vi "Get comma separated item from string.vi"(7 "Field separator (comma)":string=",", 8 "error in (no error)":errorcluster, 9 "Field Num (1-n)":u32, 10 "Preamble to first item":string, 11 "String to parse with commas":string) -> (0 "error out":errorcluster, 3 "Item string value":string)   [LabVIEW 2024]
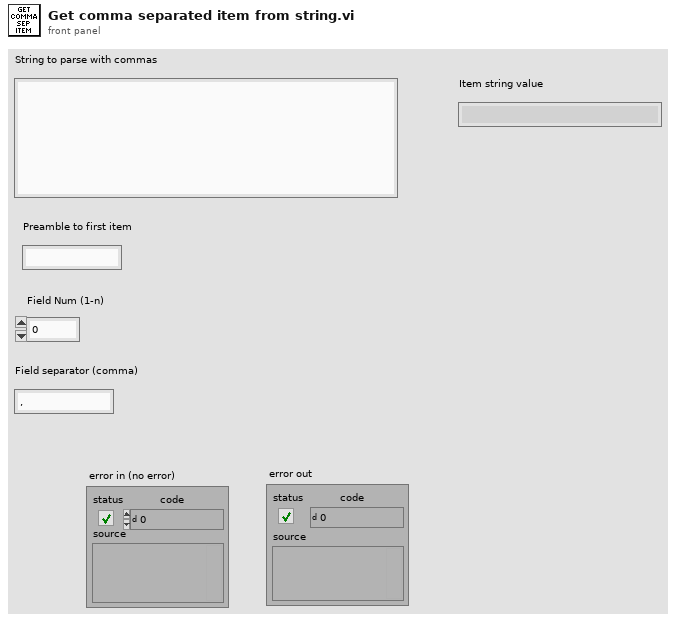
[diagram p1: front panel]
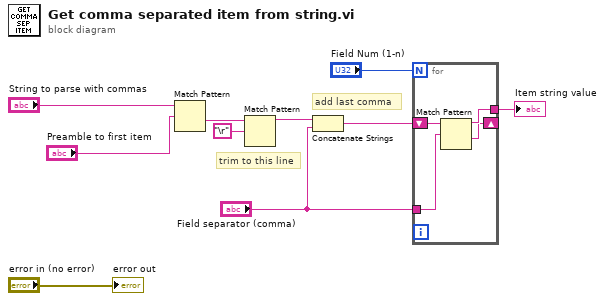
[diagram p0: block diagram]
diagram:
  # "add last comma"
  # "trim to this line"
  n1 = Match Pattern(string="String to parse with commas", regular expression="Preamble to first item") -> (after substring=w7:string)  [unwired: 1 in, 3 out]
  n2 = Match Pattern(string=w7, regular expression="\r") -> (before substring=w5:string)  [unwired: 1 in, 3 out]
  n3 = Concatenate Strings(w5, "Field separator (comma)") -> (w4:string)
  n4 = for {
    N: "Field Num (1-n)" -> [_]
    shift-right: [w12] -> _
    shift-left: w4 -> [w14]
    tunnel: [w13] -> w3
    tunnel: "Field separator (comma)" -> [w11]
    n5 = Match Pattern(string=w14, regular expression=w11) -> (before substring=w13:string, after substring=w12:string)  [unwired: 1 in, 2 out]
  }
  "Item string value" <- w3
  "error out" <- "error in (no error)"
